vi "LIN Laden Polynom setzen.vi"(3 "Span Iindex":i32, 5 "Settings Cluster old":T15, 7 "Setup Daten-Cluster old":T16, 8 "error in (no error)":errorcluster caption="Fehler (Eingang, kein Fehler)", 9 "LIN Protokoll Daten":T1 {"zusätzliche Zeitdauer Erster Punkt" format="%#_5g"; "Lin Modus" items=["Cal Gas to PNS", "Cal Gas to Samplepoint", "Measure"]; "Gas Ablaufdatum" format="%<%d.%m.%Y>T"; "HovaCAL Flow AutoLin"."HovaCAL Flow Input Cluster" format="%.2f"; "Gasflasche" items=["----"=10000, "IAG MG"=0, "IAG NH3 3000"=1, "IAG NH3 2000"=2, "IAG NH3 200"=3]; "Conditions:" items=["field", "laboratory"]; "Kalibrierauswahl" items=["Inaktiv", "Aktiv"]; "Anzahl Stufen" format="%#_5g"; "Zeitdauer Stufe" format="%#_5g"; "Verdünnungsgas" items=["N2", "O2"]; "Komponentenauswahl"."Konzentration" format="%#.6f"; "Gasnummer:" min=1 max=5; "Prüfgas Konzentration" format="%#.6f"; "Polynomkoeff." format="%#_18f"}, 10 "Setup Daten-Cluster new":T16, 11 "Settings Cluster new":T15) -> (0 "error out":errorcluster caption="Fehler (Ausgang)")   [LabVIEW 2020, in "Linearisierung v2.lvlib"]
uses:
  Linearisierung v2.lvlib
  SpanEinstellungen/LIN Loading Setup Data.ctl
  Lin-Polynom Daten.ctl
  KomponentenArray.ctl
  Visualisierungs Elemente/Auswahlfeld.ctl
  Visualisierungs Elemente/Zahlen-Eingabefeld.ctl
  EPA Optionsfeld.ctl
  Gasteiler/HovaCal/AutoLin Hovacal.ctl
  Kalibrieroption.ctl
  EPA1065-307/Condition.ctl
  Seiten/System Einstellungen V2/Konfig Gasflasche.ctl
  Seiten/System Einstellungen V2/Gasflasche Auswahl.ctl
  Gasteiler/HovaCAL_Interface/Controls/Flow Einstellung.ctl
  Gasteiler/HovaCAL_Interface/Controls/Pump state.ctl
  Seiten/CalGas Aufschaltung/Lin Modus.ctl
  Aktion Lin Daten aufarbeiten.ctl
  Auswahl Polynom Ordnung.ctl
  Protokoll/Protokoll.lvlib
  SpanEinstellungen/SpanEinstellungen.lvlib
  Gasteiler/Gasteiler.lvlib
  Gasteiler/HovaCal/HovaCal.lvlib
  EPA1065-307/Linearity verification 1065-307.lvlib
  Seiten/System Einstellungen V2/System Einstellungen V2.lvlib
  Gasteiler/HovaCAL_Interface/Controls/Controls.lvlib
  Seiten/CalGas Aufschaltung/CalGas Aufschaltung.lvlib
panel:
  out "LIN Protokoll Daten out":T1 {"zusätzliche Zeitdauer Erster Punkt" format="%#_5g"; "Lin Modus" items=["Cal Gas to PNS", "Cal Gas to Samplepoint", "Measure"]; "Gas Ablaufdatum" format="%<%d.%m.%Y>T"; "HovaCAL Flow AutoLin"."HovaCAL Flow Input Cluster" format="%.2f"; "Gasflasche" items=["----"=10000, "IAG MG"=0, "IAG NH3 3000"=1, "IAG NH3 2000"=2, "IAG NH3 200"=3]; "Conditions:" items=["field", "laboratory"]; "Kalibrierauswahl" items=["Inaktiv", "Aktiv"]; "Anzahl Stufen" format="%#_5g"; "Zeitdauer Stufe" format="%#_5g"; "Verdünnungsgas" items=["N2", "O2"]; "Komponentenauswahl"."Konzentration" format="%#.6f"; "Gasnummer:" min=1 max=5; "Prüfgas Konzentration" format="%#.6f"; "Polynomkoeff." format="%#_18f"}
  # "%"
  # "%"
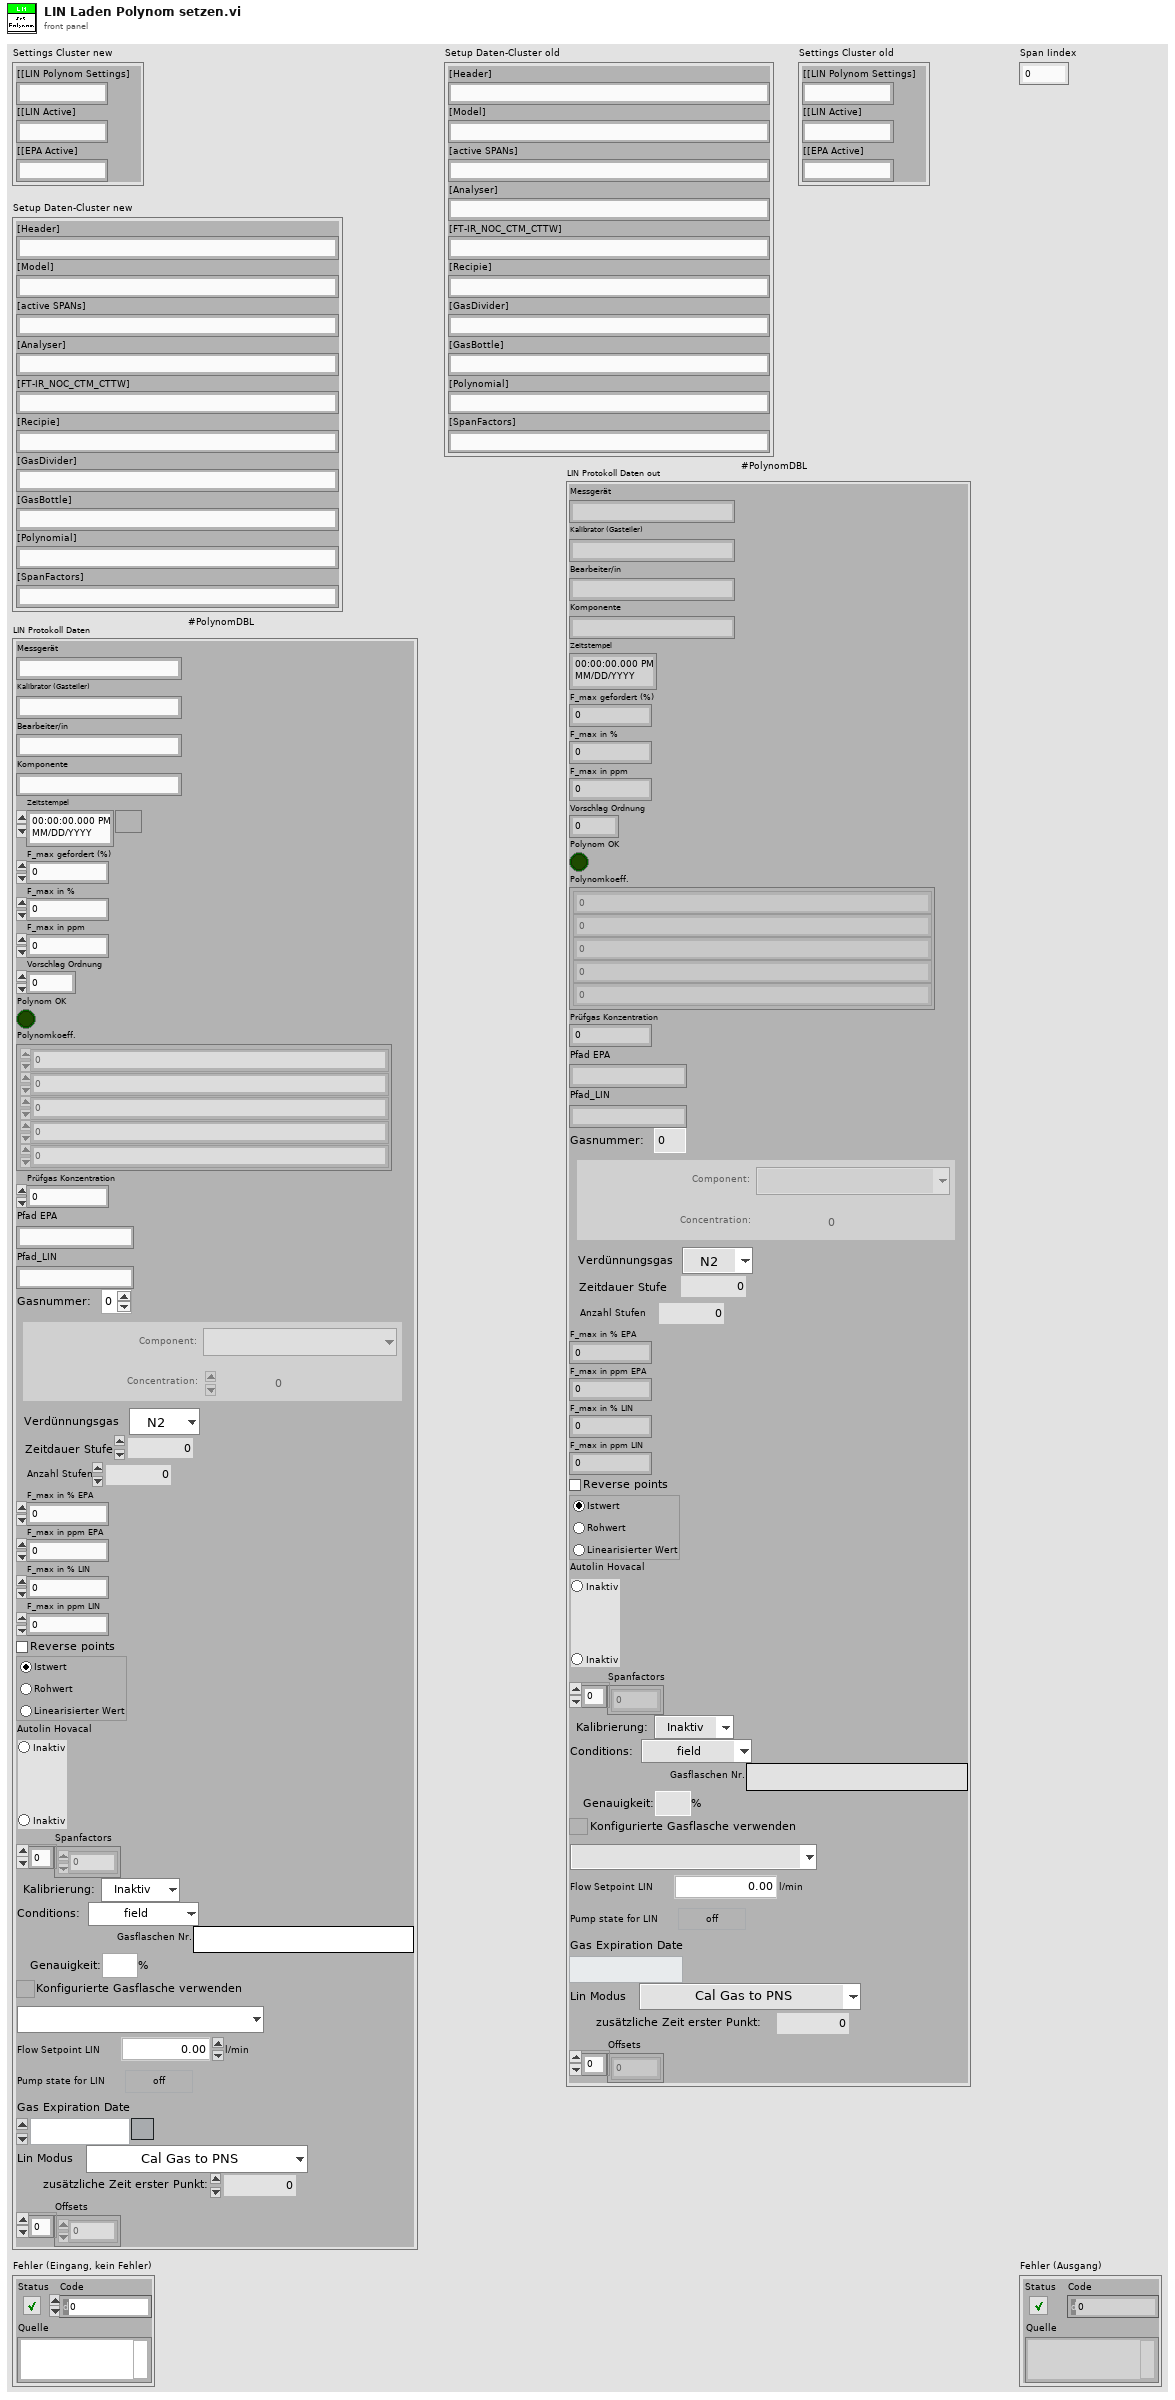
[diagram p1: front panel]
types:
  T1 = typedef "Linearisierung v2.lvlib/Lin-Polynom Daten.ctl" = cluster{"Messgerät":string, "Kalibrator (Gasteiler)":string, "Bearbeiter/in":string, "Komponente":string, "Zeitstempel":timestamp, "F_max gefordert (%)":sgl, "F_max in %":sgl, "F_max in ppm":sgl, "Vorschlag Ordnung":i32, "Polynom OK":bool, "Polynomkoeff.":dbl[], "Prüfgas Konzentration":dbl, "Pfad EPA":string, "Pfad_LIN":string, "Gasnummer:":u8, "Komponentenauswahl":T2, "Verdünnungsgas":T4, "Zeitdauer Stufe":T5, "Anzahl Stufen":T5, "F_max in % EPA":sgl, "F_max in ppm EPA":sgl, "F_max in % LIN":sgl, "F_max in ppm LIN":sgl, "Punkte umkehren":bool, "EPA Optionsfeld":T6, "Autolin Hovacal":T7, "Spanfactors":sgl[], "Kalibrierauswahl":T8, "Conditions:":T9, "Gasflaschen Nr.:":string, "Bottle Accuracy":dbl, "Konfig Gasflasche":T10, "Gasflasche":T11, "HovaCAL Flow AutoLin":T12, "MFC Output":T13, "Gas Ablaufdatum":timestamp, "Lin Modus":T14, "zusätzliche Zeitdauer Erster Punkt":sgl, "Offsets":sgl[]}
  T2 = typedef "Linearisierung v2.lvlib/KomponentenArray.ctl" = cluster{"Komponente:":T3, "Konzentration":dbl}[]
  T3 = typedef "Auswahlfeld.ctl" = u16
  T4 = typedef "Linearisierung v2.lvlib/Gasteiler.lvlib/Prüfgas in.ctl" = u16
  T5 = typedef "Zahlen-Eingabefeld.ctl" = sgl
  T6 = typedef "Linearisierung v2.lvlib/EPA Optionsfeld.ctl" = enum32{"Istwert", "Rohwert", "Linearisierter Wert"}
  T7 = typedef "Linearisierung v2.lvlib/Gasteiler.lvlib/HovaCal.lvlib/AutoLin Hovacal.ctl" = enum32{"Keine Auswahl", "Optionsauswahl 1", "Optionsauswahl 2"}
  T8 = typedef "Linearisierung v2.lvlib/Kalibrieroption.ctl" = u16
  T9 = typedef "Linearisierung v2.lvlib/Linearity verification 1065-307.lvlib/Condition.ctl" = u16
  T10 = typedef "System Einstellungen V2.lvlib/Konfig Gasflasche.ctl" = bool
  T11 = typedef "System Einstellungen V2.lvlib/Gasflasche Auswahl.ctl" = u16
  T12 = typedef "Linearisierung v2.lvlib/Gasteiler.lvlib/HovaCAL_Interface.lvlib/Controls.lvlib/Flow Einstellung.ctl" = cluster{"HovaCAL Flow Input Cluster":dbl}
  T13 = typedef "Linearisierung v2.lvlib/Gasteiler.lvlib/HovaCAL_Interface.lvlib/Controls.lvlib/Pump state.ctl" = cluster{"Run":bool}
  T14 = typedef "CalGas Aufschaltung.lvlib/Lin Modus.ctl" = u16
  T15 = cluster{"[[LIN Polynom Settings]":string, "[[LIN Active]":string, "[[EPA Active]":string}
  T16 = typedef "Linearisierung v2.lvlib/SpanEinstellungen.lvlib/LIN Loading Setup Data.ctl" = cluster{"[Header]":string, "[Model]":string, "[active SPANs]":string, "[Analyser]":string, "[FT-IR_NOC_CTM_CTTW]":string, "[Recipie]":string, "[GasDivider]":string, "[GasBottle]":string, "[Polynomial]":string, "[SpanFactors]":string}
  T17 = cluster{"Komponente:":u16, "Konzentration IST":dbl}[]
  T18 = typedef "Linearisierung v2.lvlib/Protokoll.lvlib/Aktion LIN Polynom Ordnung je Komponente für Protokoll.ctl" = enum16{"lesen", "schreiben", "init", "schreiben viewonly", "init initial"}
  T19 = typedef "Linearisierung v2.lvlib/Aktion Lin Daten aufarbeiten.ctl" = enum16{"lesen", "Protkolldaten", "speichern", "laden", "EPA auswerten", "Tabelle schreiben", "Lin auswerten", "Tab init", "Stufentabelle", "EPA aktiviert", "Nachbehandlung laden", "Tabelle löschen", "Istwerte löschen", "Zeile löschen", "Zeile einfügen", "LIN aktiviert", "LIN/EPA aktiv laden", "EGAK Tab", "LIN übernehmen", "Tab init ohne Stufen"}
  T20 = typedef "Linearisierung v2.lvlib/Auswahl Polynom Ordnung.ctl" = enum16{"autom.", "raw", "actual", "1", "2", "3", "4"}
  T21 = cluster{"active SPAN Idx":i32, "active Component Index":i32}
  T22 = typedef "Linearisierung v2.lvlib/Eingabetabelle.ctl" = string[][]
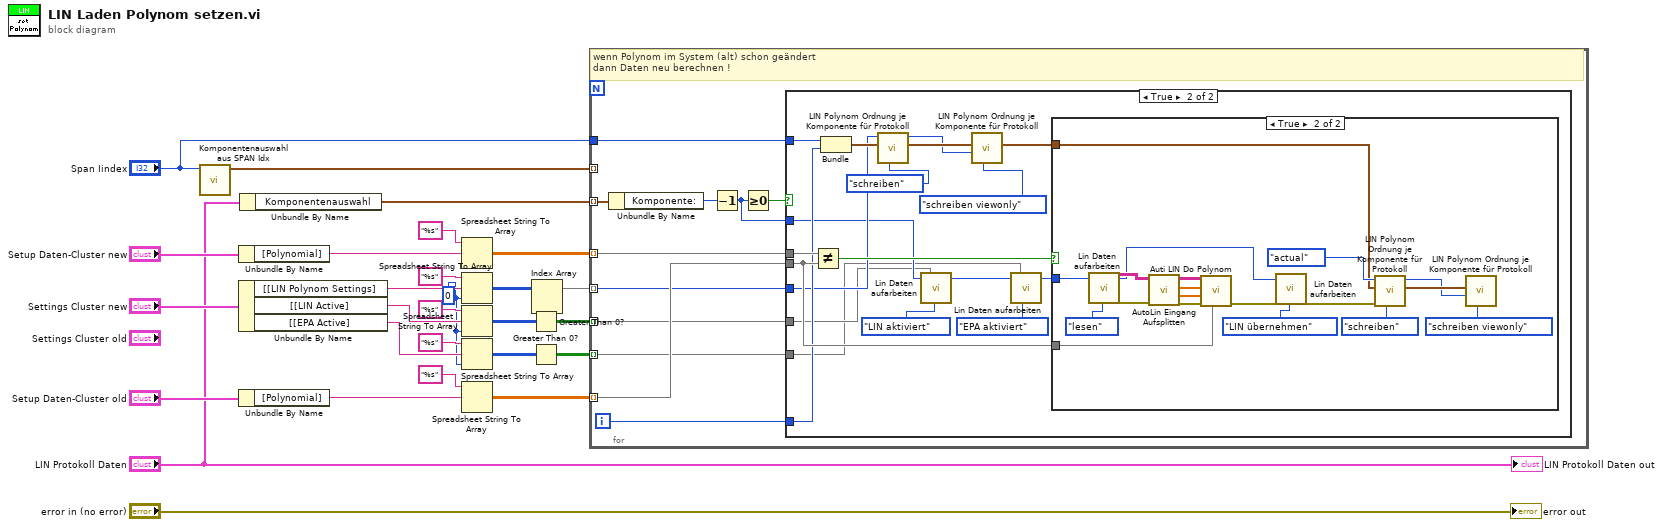
[diagram p0: block diagram]
diagram:
  w7 = u16 0
  n1 = call "Komponentenauswahl aus SPAN Idx.vi"("Span Iindex"="Span Iindex") -> ("Komponentenauswahl"=w16:T17)  [unwired: 9 in, 1 out]
  n2 = Unbundle By Name("Setup Daten-Cluster new") -> ("[Polynomial]"=w23:string)
  n3 = Unbundle By Name("Settings Cluster new") -> ("[[LIN Polynom Settings]"=w13:string, "[[LIN Active]"=w11:string, "[[EPA Active]"=w8:string)
  n4 = Unbundle By Name("Setup Daten-Cluster old") -> ("[Polynomial]"=w20:string)
  n5 = Unbundle By Name("LIN Protokoll Daten") -> ("Komponentenauswahl"=w17:T2)
  n6 = Spreadsheet String To Array(format string="%s" ("Format-String"), spreadsheet string=w23) -> (array=w19:dbl[][])  [unwired: 2 in]
  n7 = Spreadsheet String To Array(format string="%s" ("Format-String"), spreadsheet string=w13, array type (2D Dbl)=w7) -> (array=w2:u16[][])  [unwired: 1 in]
  n8 = Spreadsheet String To Array(format string="%s" ("Format-String"), spreadsheet string=w11, array type (2D Dbl)=w7) -> (array=w6:u16[][])  [unwired: 1 in]
  n9 = Spreadsheet String To Array(format string="%s" ("Format-String"), spreadsheet string=w8, array type (2D Dbl)=w7) -> (array=w5:u16[][])  [unwired: 1 in]
  n10 = Spreadsheet String To Array(format string="%s" ("Format-String"), spreadsheet string=w20) -> (array=w9:dbl[][])  [unwired: 2 in]
  n11 = Greater Than 0?(x=w6) -> (x > 0?=w4:bool[][])
  n12 = Greater Than 0?(x=w5) -> (x > 0?=w3:bool[][])
  n13 = Index Array(array=w2) -> (element=w1:u16[])  [unwired: 2 in]
  n14 = for {
    tunnel: w19 -> [w35] mode=indexing
    tunnel: w9 -> [w34] mode=indexing
    tunnel: w17 -> [w38] mode=indexing
    tunnel: w16 -> [_] mode=indexing
    tunnel: "Span Iindex" -> [w32]
    tunnel: w4 -> [w29] mode=indexing
    tunnel: w3 -> [w28] mode=indexing
    tunnel: w1 -> [w30] mode=indexing
    i -> [w31]
    # "wenn Polynom im System (alt) schon geändert\ndann Daten neu berechnen !"
    n15 = Unbundle By Name(w38) -> ("Komponente:"=w37:T3)
    n16 = Decrement(x=w37) -> (x-1=w33:T3)
    n17 = Greater Or Equal To 0?(x=w33) -> (x >= 0?=w36:bool)
    n18 = case shown="True" w36 {
      tunnel: w35 -> [_ w57]
      tunnel: w34 -> [_ w55]
      tunnel: w33 -> [_ w48]
      tunnel: w32 -> [_ w53]
      tunnel: w31 -> [_ w54]
      tunnel: w30 -> [_ w50]
      tunnel: w29 -> [_ w47]
      tunnel: w28 -> [_ w43]
      frame False {
      }
      frame True {
        n19 = Not Equal?(x=w57, y=w55) -> (x != y?=w56:bool)
        n20 = Bundle("Span Iindex"=w53, w54) -> (w51:cluster{"Span Iindex":i32, i32})  [unwired: 1 in]
        n21 = call "LIN Polynom Ordnung je Komponente für Protokoll.vi"("Aktion"=Aktion_LIN_Polynom_Ordnung_je_Komponente_für_Protokoll."schreiben", "Index in"=w51, "Polynom-Ordnung"=w50) -> ("Index out"=w41:T21, "Polynom-Ordnung out"=w39:T20)  [unwired: 2 in, 5 out]
        n22 = call "Lin Daten aufarbeiten.vi"("Index (Seite)"=w48, "Aktiv"=w47, "Aktionen"=Aktion_Lin_Daten_aufarbeiten."LIN aktiviert") -> ("Index (Seite) out"=w46:i32)  [unwired: 14 in, 10 out]
        n23 = call "LIN Polynom Ordnung je Komponente für Protokoll.vi"("Aktion"=Aktion_LIN_Polynom_Ordnung_je_Komponente_für_Protokoll."schreiben viewonly", "Polynom-Ordnung view only"=w39, "Index in"=w41) -> ("Index out"=w40:T21)  [unwired: 2 in, 6 out]
        n24 = call "Lin Daten aufarbeiten.vi"("Index (Seite)"=w46, "Aktiv"=w43, "Aktionen"=Aktion_Lin_Daten_aufarbeiten."EPA aktiviert") -> ("Index (Seite) out"=w45:i32)  [unwired: 14 in, 10 out]
        n25 = case shown="True" w56 {
          tunnel: w55 -> [_ w67]
          tunnel: w45 -> [_ w66]
          tunnel: w40 -> [_ w61]
          frame False {
          }
          frame True {
            n26 = call "Lin Daten aufarbeiten.vi"("Index (Seite)"=w66, "Aktionen"=Aktion_Lin_Daten_aufarbeiten."lesen") -> ("Eingabetabelle"=w69:T22, "Index (Seite) out"=w65:i32, "error out"=w68:errorcluster)  [unwired: 15 in, 8 out]
            n27 = call "AutoLin Eingang Aufsplitten.vi"("error in (no error)"=w68, "Eingabetabelle"=w69) -> ("error out"=w71:errorcluster, "Sollwerte"=w72:dbl[], "Rohwerte"=w73:dbl[], "Eingabetabelle out"=w74:T22)  [unwired: 5 in, 1 out]
            n28 = call "Auti LIN Do Polynom.vi"("Polynomkoeff."=w67, "error in (no error)"=w71, "Sollwerte"=w72, "Rohwerte"=w73, "Eingabetabelle"=w74) -> ("error out"=w64:errorcluster)  [unwired: 4 in, 2 out]
            n29 = call "Lin Daten aufarbeiten.vi"("Index (Seite)"=w65, "error in (no error)"=w64, "Aktionen"=Aktion_Lin_Daten_aufarbeiten."LIN übernehmen") -> ("error out"=w62:errorcluster)  [unwired: 14 in, 10 out]
            n30 = call "LIN Polynom Ordnung je Komponente für Protokoll.vi"("Aktion"=Aktion_LIN_Polynom_Ordnung_je_Komponente_für_Protokoll."schreiben", "error in (no error)"=w62, "Index in"=w61, "Polynom-Ordnung"=Auswahl_Polynom_Ordnung."actual") -> ("Index out"=w59:T21, "Polynom-Ordnung out"=w58:T20)  [unwired: 1 in, 5 out]
            n31 = call "LIN Polynom Ordnung je Komponente für Protokoll.vi"("Aktion"=Aktion_LIN_Polynom_Ordnung_je_Komponente_für_Protokoll."schreiben viewonly", "Polynom-Ordnung view only"=w58, "Index in"=w59) -> ()  [unwired: 2 in, 7 out]
          }
        }
      }
    }
  }
  "error out" <- "error in (no error)"
  "LIN Protokoll Daten out" <- "LIN Protokoll Daten"
